vi "BR Update Data.vi"(0 "AJ Run in":T1) -> (1 "appended array":string[](array[string]), 5 "AJ Run":T1)   [LabVIEW 2014]
uses:
  Type'def/AJ_RunTable.ctl
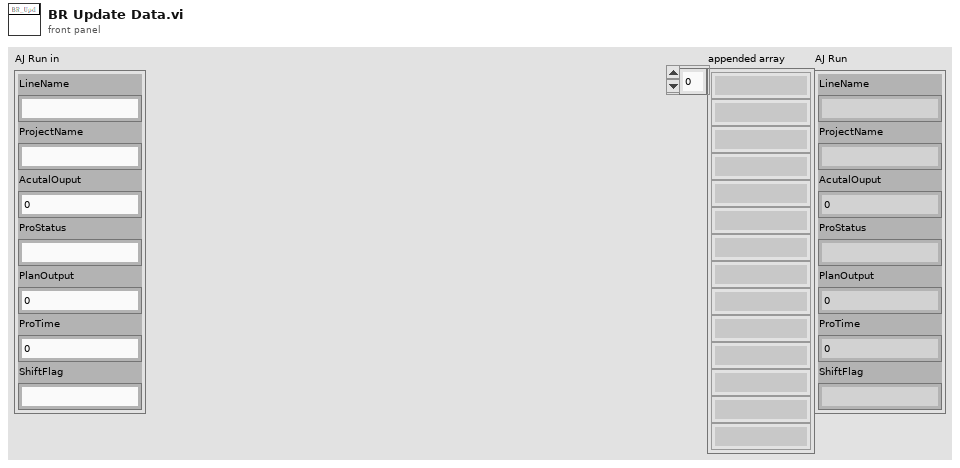
[diagram p1: front panel]
types:
  T1 = typedef "AJ_RunTable.ctl" = cluster{"LineName":string, "ProjectName":string, "AcutalOuput":u32, "ProStatus":string, "PlanOutput":u32, "ProTime":u32, "ShiftFlag":string}
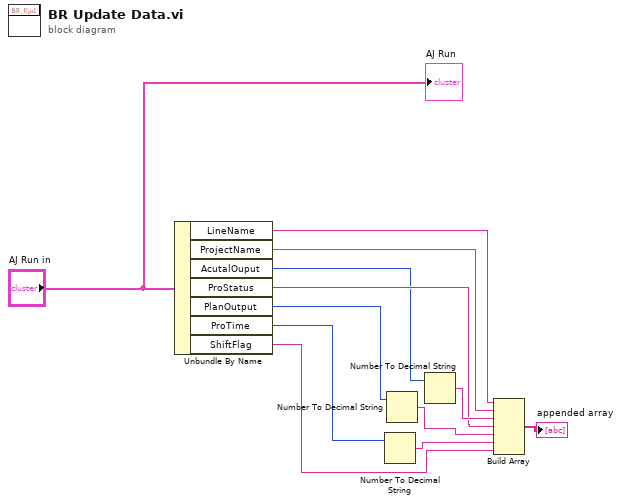
[diagram p0: block diagram]
diagram:
  n1 = Unbundle By Name("AJ Run in") -> ("LineName"=w9:string, "ProjectName"=w8:string, "AcutalOuput"=w1:u32, "ProStatus"=w6:string, "PlanOutput"=w7:u32, "ProTime"=w4:u32, "ShiftFlag"=w2:string)
  n2 = Number To Decimal String(number=w4) -> (decimal integer string=w3:string)  [unwired: 1 in]
  n3 = Number To Decimal String(number=w7) -> (decimal integer string=w5:string)  [unwired: 1 in]
  n4 = Number To Decimal String(number=w1) -> (decimal integer string=w12:string)  [unwired: 1 in]
  n5 = Build Array(w9, w8, w12, w6, w5, w3, w2) -> (→"appended array":string[])
  "AJ Run" <- "AJ Run in"
